vi "Get Node Wild.vi"(8 "error in (no error)":errorcluster, 10 "Path":string, 11 "Tree in":refnum<class "Tree.lvclass">) -> (0 "error out":errorcluster, 2 "Node array out":refnum<class "TreeNodeArray.lvclass">, 3 "Tree out":refnum<class "Tree.lvclass">)   [LabVIEW 2012, in "MDSplus.lvlib" / "Tree.lvclass"]
uses:
  <vilib>/MDSplus/Classes/Tree_Class/Tree.lvclass
  <vilib>/MDSplus/Classes/TreeNodeArray_Class/TreeNodeArray.lvclass
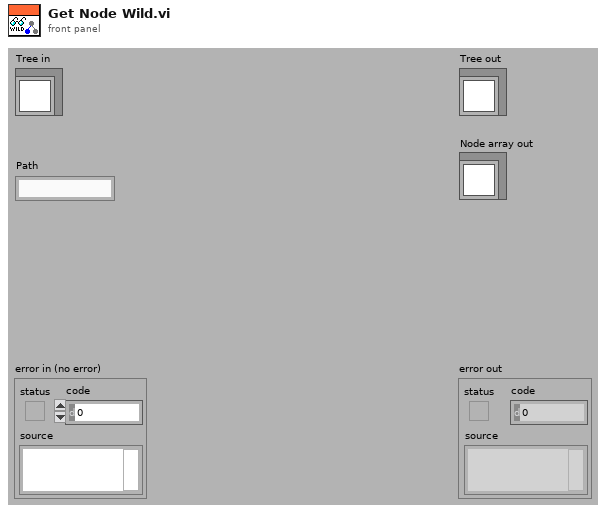
[diagram p1: front panel]
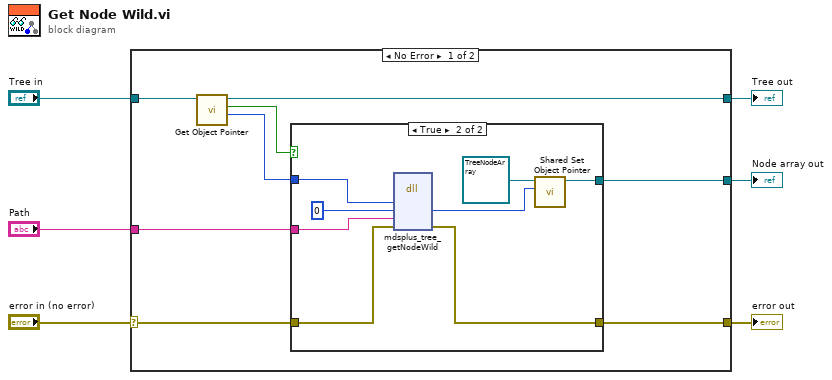
[diagram p0: block diagram]
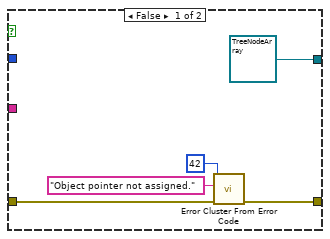
[diagram p2: hidden frame]
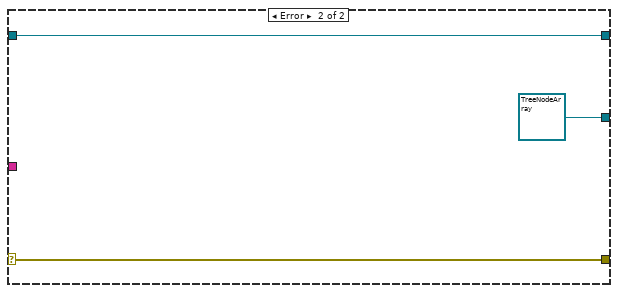
[diagram p3: hidden frame]
diagram:
  n1 = case shown="No Error" "error in (no error)" {
    selector: "error in (no error)" -> [w8 w30]
    tunnel: [w7 w30] -> w5
    tunnel: [w13 w29] -> w3
    tunnel: "Tree in" -> [w14 w29]
    tunnel: "Path" -> [w12 _]
    tunnel: [w11 refnum<class "TreeNodeArray.lvclass"> refnum ("TreeNode out")] -> w1
    frame No Error {
      n2 = call-dynamic "Get Object Pointer.vi"("Tree in"=w14) -> ("Object Pointer"=w9:i64, "Assigned object pointer?"=w10:bool, "Tree out"=w13:refnum<class "Tree.lvclass">)  [unwired: 8 in]
      n3 = case shown="True" w10 {
        tunnel: w12 -> [_ w26]
        tunnel: [refnum<class "TreeNodeArray.lvclass"> refnum ("Data out") w23] -> w11
        tunnel: w9 -> [_ w22]
        tunnel: w8 -> [w16 w21]
        tunnel: [w15 w20] -> w7
        frame False {
          n4 = call <vilib>:"Error Cluster From Error Code.vi"("error in (no error)"=w16, "error message (\"\")"="Object pointer not assigned." ("error message (\"\")"), "error code (0)"=42) -> ("error out"=w15:errorcluster)  [unwired: 6 in]
        }
        frame True {
          n5 = dll-call lib="MDSobjectsLVShr" fn="mdsplus_tree_getNodeWild"("lvTreePtr"=w22, "lvTreeNodeArrayPtrOut"=i64 0 ("lvTreeNodePtr"), "pathIn"=w26, "error"=w21) -> ("lvTreeNodeArrayPtrOut"=w24:i64, "error"=w20:errorcluster)  [unwired: 6 in, 2 out]
          n6 = call <vilib>:"Shared Set Object Pointer.vi"("Object Pointer"=w24, "TreeNodeArray in"=refnum<class "TreeNodeArray.lvclass"> refnum ("TreeNode")) -> ("TreeNodeArray out"=w23:refnum<class "TreeNodeArray.lvclass">)  [unwired: 9 in]
        }
      }
    }
    frame Error {
    }
  }
  "error out" <- w5
  "Tree out" <- w3
  "Node array out" <- w1
